vi "Bounds.vi"(1 "XRef":refnum<vi>, 2 "State In":T2={"Input Type"=variant(dbl 0.0), "Width"=0, "Typedef Name"="", "Value Type"=variant, "Selection"=0, "Options"=[], "Selections"=[], "Display Selections"=[], "Element Names"=[], "Typedef Name Width"=0, "Display Selection Width"=[], "Code Generated"=FALSE}) -> (0 "Bounds":cluster{"Width":T1, "Height":T1})   [LabVIEW 2015, in "Read-Write-Signals.xnode"]
doc: "This ability VI is used to tell LabVIEW your current bounds. If you want to update your bounds, you must inform LabVIEW through the UpdateImageAndBounds reply of another ability VI. If you change your bounds, you will also probably want to update your image.\n\nDefault behavior: None.\n\nThis ability does not provide UI and OS messages are not handled."
uses:
  Read-Write-Signals.xnode
  State.ctl
  Read-Write-Signals Item.ctl
  Read-Write-Signals Sub Item.ctl
  Read-Write-Signals Sub Item Type.ctl
  Read-Write-Signals Selection.ctl
  Read-Write-Signals Display Selection.ctl
  <vilib>/XNodeSupport/XNodeInt.ctl
  <vilib>/XNodeSupport/NI_XNodeSupport.lvlib
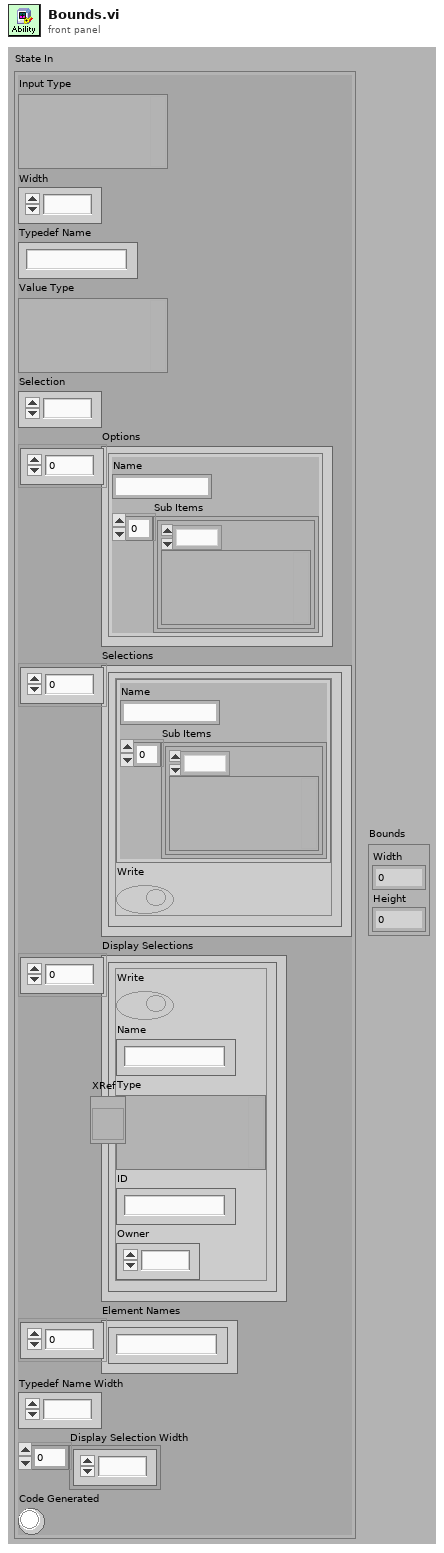
[diagram p1: front panel]
types:
  T1 = typedef "NI_XNodeSupport.lvlib/XNodeInt.ctl" = i32
  T2 = typedef "Read-Write-Signals.xnode/State.ctl" = cluster{"Input Type":variant, "Width":i32, "Typedef Name":string, "Value Type":variant, "Selection":i32, "Options":T3[], "Selections":T6[], "Display Selections":T7[], "Element Names":string[], "Typedef Name Width":i32, "Display Selection Width":i32[], "Code Generated":bool}
  T3 = typedef "Read-Write-Signals Item.ctl" = cluster{"Name":string, "Sub Items":T4[]}
  T4 = typedef "Read-Write-Signals Sub Item.ctl" = cluster{"Type":T5, "Value":variant}
  T5 = typedef "Read-Write-Signals Sub Item Type.ctl" = enum8{"Cluster Element", "Array Element", "Subarray"}
  T6 = typedef "Read-Write-Signals Selection.ctl" = cluster{"Item":T3, "Write":bool}
  T7 = typedef "Read-Write-Signals Display Selection.ctl" = cluster{"Write":bool, "Name":string, "Type":variant, "ID":string, "Owner":i32}
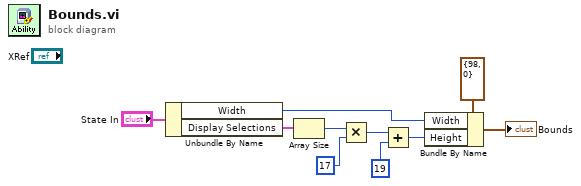
[diagram p0: block diagram]
diagram:
  n1 = Unbundle By Name("State In") -> ("Width"=w4:i32, "Display Selections"=w3:T7[])
  n2 = Array Size(array=w3) -> (size(s)=w5:i32)
  n3 = Multiply(x=w5, y=17) -> (x*y=w10:i32)
  n4 = Add(x=w10, y=19) -> (x+y=w7:i32)
  n5 = Bundle By Name(cluster=cluster{"Width":T1, "Height":T1} {"Width"=98, "Height"=0} ("Bounds"), "Width"=w4, "Height"=w7) -> (→"Bounds":cluster{"Width":T1, "Height":T1})
